vi "PID setting FGV.vi"(7 "Command":T2(ring), 8 "error in (no error)":errorcluster, 10 "PID gains":T1={"proportional gain (Kc)"=0.5, "integral gain (Kc*Ts/Ti)"=0.01171875, "derivative gain (Kc*Td/Ts)"=0.01171875}, 11 "File Path":path) -> (0 "error out":errorcluster, 2 "PID gains":T1={"proportional gain (Kc)"=0.5, "integral gain (Kc*Ts/Ti)"=0.01171875, "derivative gain (Kc*Td/Ts)"=0.01171875})   [LabVIEW 2025]
doc: "This Subvi usde for CSV Initialize ,Read, Write and close.\nIntilise case; we check File avaliblity in not found create csv file\nRead Case ; Read data from csv file"
uses:
  <vilib>/Utility/file.llb/Write Delimited Spreadsheet (string).vi
  <vilib>/Utility/file.llb/Read Delimited Spreadsheet (string).vi
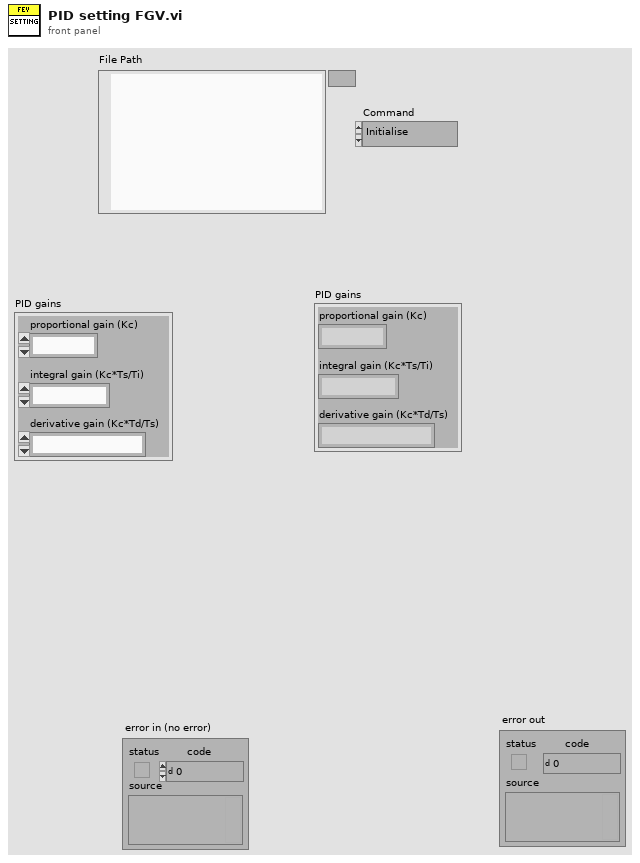
[diagram p1: front panel]
types:
  T1 = cluster{"proportional gain (Kc)":fxp<+/-,16,8>, "integral gain (Kc*Ts/Ti)":fxp<+/-,16,8>, "derivative gain (Kc*Td/Ts)":fxp<+/-,16,8>}
  T2 = enum16{"Initialise", "Read Data", "Write Data", "Close"}
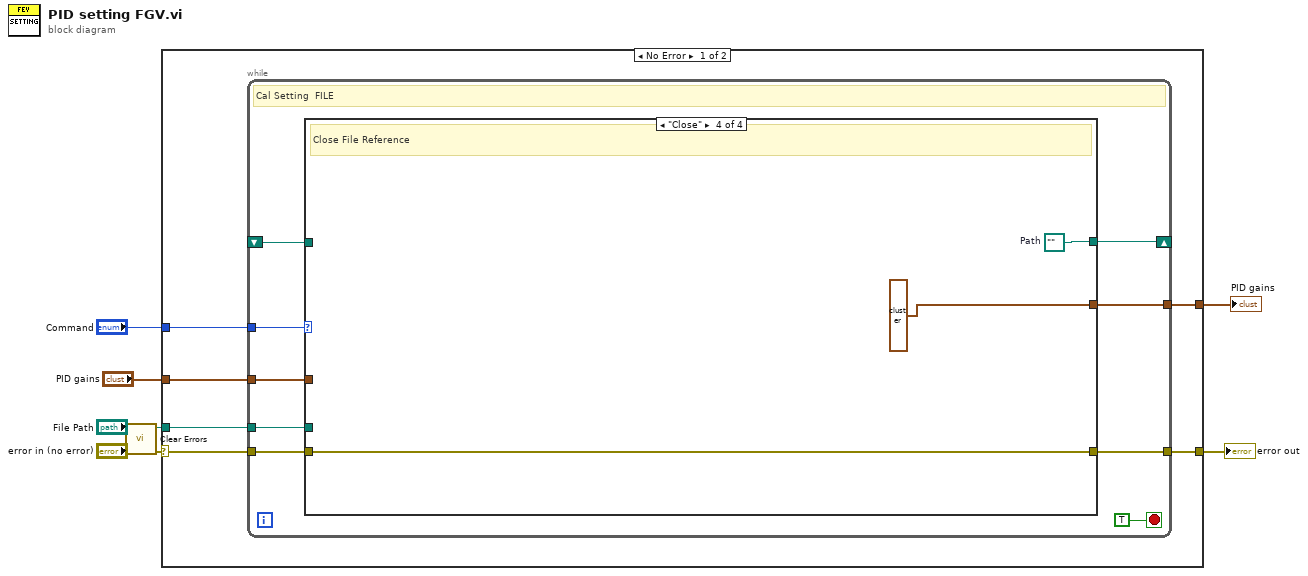
[diagram p0: block diagram]
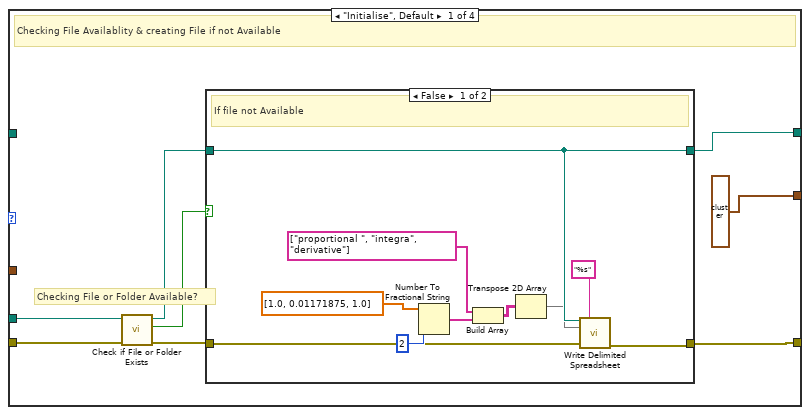
[diagram p2: hidden frame]
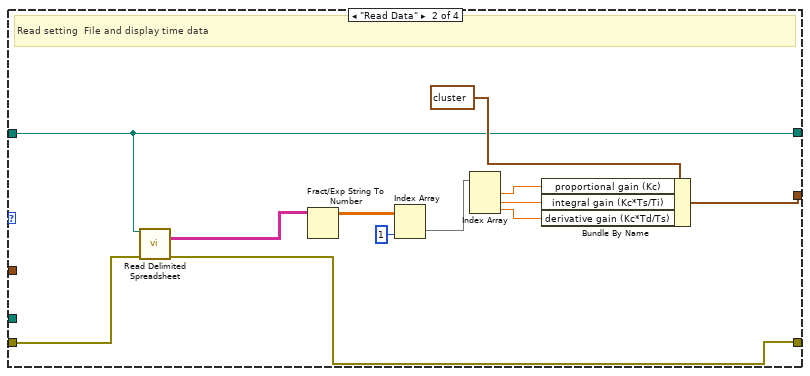
[diagram p4: hidden frame]
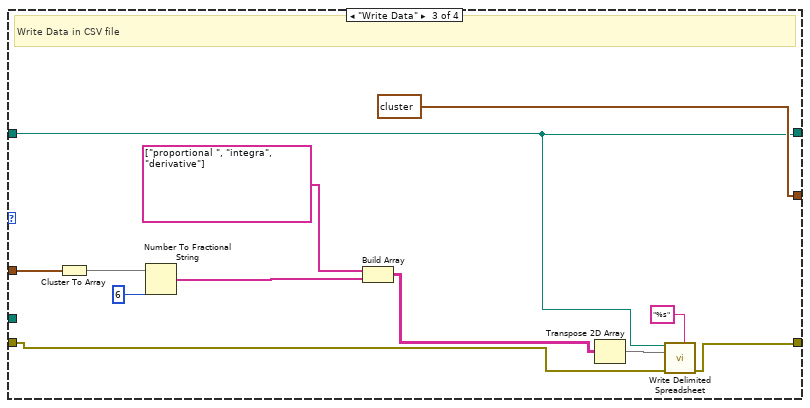
[diagram p5: hidden frame]
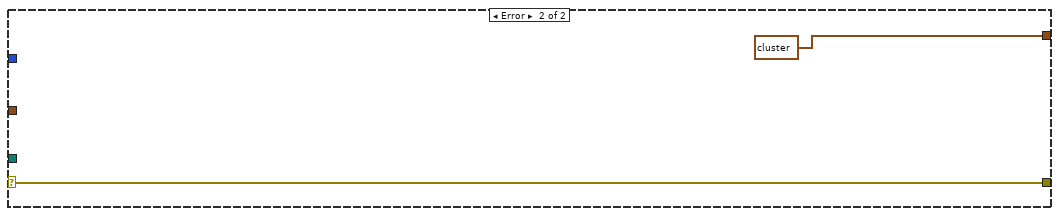
[diagram p6: hidden frame]
diagram:
  n1 = call <vilib>:"Clear Errors.vi"("error in (no error)"="error in (no error)") -> ("error out"=w1:errorcluster)  [unwired: 5 in, 1 out]
  n2 = case shown="No Error" w1 {
    selector: w1 -> [w12 w71]
    tunnel: [w11 w71] -> w6
    tunnel: "Command" -> [w13 _]
    tunnel: "File Path" -> [w10 _]
    tunnel: "PID gains" -> [w9 _]
    tunnel: [w8 T1 {"proportional gain (Kc)"=0.0, "integral gain (Kc*Ts/Ti)"=0.0, "derivative gain (Kc*Td/Ts)"=0.0} ("PID gains")] -> w2
    frame No Error {
      n3 = while {
        shift-right: [w17] -> _
        shift-left: _ -> [w16]
        tunnel: w13 -> [w21]
        tunnel: w12 -> [w20]
        tunnel: [w19] -> w11
        tunnel: w10 -> [w18]
        tunnel: w9 -> [w15]
        tunnel: [w14] -> w8
        stop <- TRUE stop-if-true
        # "Cal Setting  FILE"
        n4 = case shown="\"Close\"" w21 {
          tunnel: w20 -> [w30 w50 w58 w69]
          tunnel: [w24 w49 w57 w69] -> w19
          tunnel: w18 -> [w29 _ _ _]
          tunnel: [w27 w51 w56 w68] -> w17
          tunnel: w16 -> [_ w51 w56 _]
          tunnel: w15 -> [_ _ w66 _]
          tunnel: [T1 {"proportional gain (Kc)"=0.0, "integral gain (Kc*Ts/Ti)"=0.0, "derivative gain (Kc*Td/Ts)"=0.0} ("PID gains") w52 T1 {"proportional gain (Kc)"=0.0, "integral gain (Kc*Ts/Ti)"=0.0, "derivative gain (Kc*Td/Ts)"=0.0} ("PID gains") T1 {"proportional gain (Kc)"=0.0, "integral gain (Kc*Ts/Ti)"=0.0, "derivative gain (Kc*Td/Ts)"=0.0} ("PID gains")] -> w14
          frame "Initialise", Default {
            # "Checking File or Folder Available?"
            # "Checking File Availablity & creating File if not Available"
            n5 = call <vilib>:"Check if File or Folder Exists.vi"("error in (no error)"=w30, "path"=w29) -> ("error out"=w25:errorcluster, "file or folder exists?"=w28:bool, "dup path"=w26:path)  [unwired: 7 in]
            n6 = case shown="False" w28 {
              tunnel: [w35 w42] -> w27
              tunnel: w26 -> [w35 w42]
              tunnel: w25 -> [w32 w41]
              tunnel: [w31 w41] -> w24
              frame False {
                # "If file not Available"
                n7 = Number To Fractional String(number=dbl[] [1.0, 0.01171875, 1.0], precision (6)=i16 2) -> (F-format string=w39:string[])  [unwired: 2 in]
                n8 = Build Array(string[] ["proportional ", "integra", "derivative"] ("element"), w39) -> (w40:string[][])
                n9 = Transpose 2D Array(2D array=w40) -> (transposed array=w34:string[][])
                n10 = call-poly <vilib>:"Write Delimited Spreadsheet.vi"("file path (dialog if empty)"=w35, "format (%s)"="%s", "2D data"=w34, "error in (no error)"=w32) -> ("error out"=w31:errorcluster)  [unwired: 10 in, 1 out]
              }
              frame True {
                # "If File available"
              }
            }
          }
          frame "Read Data" {
            # "Read setting  File and display time data"
            n11 = call-poly <vilib>:"Read Delimited Spreadsheet.vi"("file path (dialog if empty)"=w51, "error in (no error)"=w50) -> ("all rows"=w47:string[][], "error out"=w49:errorcluster)  [unwired: 8 in, 4 out]
            n12 = Fract/Exp String To Number(string=w47) -> (number=w46:dbl[][])  [unwired: 3 in, 1 out]
            n13 = Index Array(array=w46, index (col)=1 ("disabled index (col)")) -> (element=w48:dbl[])  [unwired: 1 in]
            n14 = Index Array(array=w48) -> (element #1=w45:dbl, element #2=w44:dbl, element #3=w43:dbl)  [unwired: 3 in]
            n15 = Bundle By Name(cluster=T1 {"proportional gain (Kc)"=0.0, "integral gain (Kc*Ts/Ti)"=0.0, "derivative gain (Kc*Td/Ts)"=0.0} ("PID gains"), "proportional gain (Kc)"=w45, "integral gain (Kc*Ts/Ti)"=w44, "derivative gain (Kc*Td/Ts)"=w43) -> (w52:T1)
          }
          frame "Write Data" {
            # "Write Data in CSV file"
            n16 = Cluster To Array(cluster=w66) -> (array=w62:fxp<+/-,16,8>[])
            n17 = Number To Fractional String(number=w62, precision (6)=i16 6) -> (F-format string=w65:string[])  [unwired: 2 in]
            n18 = Build Array(string[] ["proportional ", "integra", "derivative"] ("element"), w65) -> (w55:string[][])
            n19 = Transpose 2D Array(2D array=w55) -> (transposed array=w60:string[][])
            n20 = call-poly <vilib>:"Write Delimited Spreadsheet.vi"("file path (dialog if empty)"=w56, "format (%s)"="%s", "2D data"=w60, "error in (no error)"=w58) -> ("error out"=w57:errorcluster)  [unwired: 10 in, 1 out]
          }
          frame "Close" {
            w68 = path ""  # Path
            # "Close File Reference"
          }
        }
      }
    }
    frame Error {
    }
  }
  "error out" <- w6
  "PID gains" <- w2
